vi "data_waypoint_ref.vi"() -> ()   [LabVIEW 2018] (continued)
"Y"=530235.061300714}, {"X"=175350.88993979365, "Y"=530235.1168702191}, {"X"=175350.93419405032, "Y"=530235.1720451514}, {"X"=175350.97797018028, "Y"=530235.2272858657}, {"X"=175351.0211706906, "Y"=530235.2819733487}, {"X"=175351.06420086315, "Y"=530235.3368710969}, {"X"=175351.1069546017, "Y"=530235.391745242}, {"X"=175351.14969397328, "Y"=530235.4471543846}, {"X"=175351.19290508452, "Y"=530235.5030349332}, {"X"=175351.23708086298, "Y"=530235.5592333905}, {"X"=175351.28094664667, "Y"=530235.6163428451}, {"X"=175351.32507018273, "Y"=530235.6737500923}, {"X"=175351.36946815113, "Y"=530235.7311032579}, {"X"=175351.4141272058, "Y"=530235.7883812926}, {"X"=175351.45875193508, "Y"=530235.845434128}, {"X"=175351.5033432786, "Y"=530235.9016790844}, {"X"=175351.5477972615, "Y"=530235.9573007046}, {"X"=175351.5920627689, "Y"=530236.0123890406}, {"X"=175351.63490704828, "Y"=530236.0676302855}, {"X"=175351.67720670445, "Y"=530236.1229175301}, {"X"=175351.71963278952, "Y"=530236.1781233831}, {"X"=175351.76294240737, "Y"=530236.2322667169}, {"X"=175351.80625901482, "Y"=530236.2860770716}, {"X"=175351.84902049394, "Y"=530236.3393729797}, {"X"=175351.89089530785, "Y"=530236.3929711628}, {"X"=175351.9331973055, "Y"=530236.4457479022}, {"X"=175351.97514771618, "Y"=530236.498248212}, {"X"=175352.01617310618, "Y"=530236.5512595625}, {"X"=175352.05664432573, "Y"=530236.6049850797}, {"X"=175352.09796583082, "Y"=530236.6580865675}, {"X"=175352.13995707338, "Y"=530236.7103159536}, {"X"=175352.18166292325, "Y"=530236.7621876963}, {"X"=175352.22252090828, "Y"=530236.813099689}, {"X"=175352.26255605364, "Y"=530236.8637288735}, {"X"=175352.30208352584, "Y"=530236.9137169486}, {"X"=175352.34150491114, "Y"=530236.9634744846}, {"X"=175352.38042420865, "Y"=530237.0135842154}, {"X"=175352.4199305173, "Y"=530237.0639053108}, {"X"=175352.45956587067, "Y"=530237.114131686}, {"X"=175352.49899166732, "Y"=530237.1641844318}, {"X"=175352.53829575534, "Y"=530237.2141165627}, {"X"=175352.5774806659, "Y"=530237.2632843519}, {"X"=175352.6156511215, "Y"=530237.3132742075}, {"X"=175352.6533883326, "Y"=530237.3629312733}, {"X"=175352.6910130333, "Y"=530237.4119815769}, {"X"=175352.72911552244, "Y"=530237.4611514483}, {"X"=175352.7674107072, "Y"=530237.5110854433}, {"X"=175352.80628102296, "Y"=530237.5626092828}, {"X"=175352.84566256969, "Y"=530237.6153813166}, {"X"=175352.886305737, "Y"=530237.6688455134}, {"X"=175352.92686425932, "Y"=530237.7224420327}, {"X"=175352.96628213656, "Y"=530237.776421486}, {"X"=175353.00479581486, "Y"=530237.8295612222}, {"X"=175353.04309125987, "Y"=530237.8813875283}, {"X"=175353.0805856114, "Y"=530237.9321951261}, {"X"=175353.1178263727, "Y"=530237.9820145867}, {"X"=175353.15486826623, "Y"=530238.031681473}, {"X"=175353.19223656916, "Y"=530238.0808956837}, {"X"=175353.22936573613, "Y"=530238.1307199139}, {"X"=175353.26626025818, "Y"=530238.1808755734}, {"X"=175353.3027933256, "Y"=530238.2313119823}, {"X"=175353.33960005036, "Y"=530238.2823335917}, {"X"=175353.37707444988, "Y"=530238.3338859645}, {"X"=175353.41547161504, "Y"=530238.386566564}, {"X"=175353.45446338505, "Y"=530238.4399313043}, {"X"=175353.49378934092, "Y"=530238.4939798436}, {"X"=175353.53226842728, "Y"=530238.5480086806}, {"X"=175353.57047974097, "Y"=530238.6019472994}, {"X"=175353.60875617847, "Y"=530238.6557414449}, {"X"=175353.6469764394, "Y"=530238.7094103412}, {"X"=175353.68457545002, "Y"=530238.7638723999}, {"X"=175353.72234228044, "Y"=530238.8184738057}, {"X"=175353.76045086328, "Y"=530238.8730198212}, {"X"=175353.79898426452, "Y"=530238.9271461678}, {"X"=175353.8375490814, "Y"=530238.9808107199}, {"X"=175353.8752460613, "Y"=530239.0342536401}, {"X"=175353.91189012938, "Y"=530239.0874910104}, {"X"=175353.94910051365, "Y"=530239.1393293964}, {"X"=175353.98627210603, "Y"=530239.1909281688}, {"X"=175354.02308637538, "Y"=530239.2430096754}, {"X"=175354.05967783305, "Y"=530239.2955291213}, {"X"=175354.09668178417, "Y"=530239.3488542204}, {"X"=175354.1341990515, "Y"=530239.4023320772}, {"X"=175354.17198692198, "Y"=530239.4562597376}, {"X"=175354.20951566947, "Y"=530239.5106276667}, {"X"=175354.24727854424, "Y"=530239.5653911263}, {"X"=175354.28528886437, "Y"=530239.6202604033}, {"X"=175354.3236916914, "Y"=530239.6751662572}, {"X"=175354.36217982642, "Y"=530239.7301650902}, {"X"=175354.401261916, "Y"=530239.784725996}, {"X"=175354.4399844256, "Y"=530239.8399039346}, {"X"=175354.47800392206, "Y"=530239.8951827234}, {"X"=175354.51573281956, "Y"=530239.9501405099}, {"X"=175354.55374814585, "Y"=530240.0043061222}, {"X"=175354.5920931261, "Y"=530240.0585195966}, {"X"=175354.6307848023, "Y"=530240.1125533618}, {"X"=175354.66938268108, "Y"=530240.1672211337}, {"X"=175354.70835670453, "Y"=530240.22178347}, {"X"=175354.74747454954, "Y"=530240.2767560309}, {"X"=175354.78668856682, "Y"=530240.3322011083}, {"X"=175354.82573295297, "Y"=530240.3880961786}, {"X"=175354.86442117963, "Y"=530240.4448679785}, {"X"=175354.90385480528, "Y"=530240.5017940709}, {"X"=175354.9438868584, "Y"=530240.5585985357}, {"X"=175354.98450460396, "Y"=530240.6151670938}, {"X"=175355.02560184867, "Y"=530240.6712336912}, {"X"=175355.0663030908, "Y"=530240.7269795968}, {"X"=175355.10590519384, "Y"=530240.7830661403}, {"X"=175355.1451417851, "Y"=530240.8386587655}, {"X"=175355.1843346686, "Y"=530240.8944490728}, {"X"=175355.22404374706, "Y"=530240.9501668296}, {"X"=175355.2643191493, "Y"=530241.0056886901}, {"X"=175355.30494895973, "Y"=530241.0609420296}, {"X"=175355.34536480953, "Y"=530241.1163314045}, {"X"=175355.38549545314, "Y"=530241.1717260601}, {"X"=175355.42590157175, "Y"=530241.2271199028}, {"X"=175355.466450924, "Y"=530241.2827253059}, {"X"=175355.50749417936, "Y"=530241.3382071704}, {"X"=175355.54871472975, "Y"=530241.3943377783}, {"X"=175355.5905385754, "Y"=530241.4498939218}, {"X"=175355.6317120192, "Y"=530241.5056695165}, {"X"=175355.6725872653, "Y"=530241.5612506543}, {"X"=175355.7131346146, "Y"=530241.6170791457}, {"X"=175355.7536999294, "Y"=530241.6726922737}, {"X"=175355.79431457655, "Y"=530241.7288135714}, {"X"=175355.83564892667, "Y"=530241.7844865855}, {"X"=175355.87750007684, "Y"=530241.8402923684}, {"X"=175355.9195047443, "Y"=530241.8958912657}, {"X"=175355.96087904507, "Y"=530241.9515952377}, {"X"=175356.0021839649, "Y"=530242.0072017458}, {"X"=175356.04336760036, "Y"=530242.0628308104}, {"X"=175356.08446281333, "Y"=530242.1185134072}, {"X"=175356.1253711881, "Y"=530242.1742165342}, {"X"=175356.16642529293, "Y"=530242.2294763982}, {"X"=175356.20768692662, "Y"=530242.2839210114}, {"X"=175356.24861907747, "Y"=530242.3386751397}, {"X"=175356.28909854963, "Y"=530242.3934161742}, {"X"=175356.3297216975, "Y"=530242.4482167154}, {"X"=175356.37073719004, "Y"=530242.5026975726}, {"X"=175356.4121149016, "Y"=530242.5571573845}, {"X"=175356.45343968744, "Y"=530242.6113920517}, {"X"=175356.4948522827, "Y"=530242.6656653044}, {"X"=175356.53583169985, "Y"=530242.7208310526}, {"X"=175356.57724413514, "Y"=530242.7765537826}, {"X"=175356.61908518994, "Y"=530242.8331442699}, {"X"=175356.66122786675, "Y"=530242.8895895861}, {"X"=175356.7031677672, "Y"=530242.9460588078}, {"X"=175356.74520092676, "Y"=530243.0017108984}, {"X"=175356.78699071577, "Y"=530243.0568376329}, {"X"=175356.82860514967, "Y"=530243.1110725575}, {"X"=175356.86955351502, "Y"=530243.1650197727}, {"X"=175356.90969446828, "Y"=530243.2182091132}, {"X"=175356.9490777895, "Y"=530243.2712996902}, {"X"=175356.98857629084, "Y"=530243.3234998218}, {"X"=175357.02793550797, "Y"=530243.375025569}, {"X"=175357.06710013995, "Y"=530243.4266473373}, {"X"=175357.10620575276, "Y"=530243.4780817132}, {"X"=175357.14540980468, "Y"=530243.5298554179}, {"X"=175357.18500684414, "Y"=530243.5818288475}, {"X"=175357.2246604417, "Y"=530243.6349596942}, {"X"=175357.2641467288, "Y"=530243.6890266448}, {"X"=175357.30388953027, "Y"=530243.7438730717}, {"X"=175357.34434687858, "Y"=530243.7989260455}, {"X"=175357.38561276108, "Y"=530243.853314052}, {"X"=175357.42714635562, "Y"=530243.9080741812}, {"X"=175357.46842059385, "Y"=530243.9631946698}, {"X"=175357.50957774406, "Y"=530244.0191612169}, {"X"=175357.55071779378, "Y"=530244.0753364675}, {"X"=175357.5918336218, "Y"=530244.1320090053}, {"X"=175357.63331725454, "Y"=530244.1881499484}, {"X"=175357.6750473695, "Y"=530244.2440715226}, {"X"=175357.7166139784, "Y"=530244.2995152301}, {"X"=175357.75781324354, "Y"=530244.3550454788}, {"X"=175357.79876509352, "Y"=530244.4101791265}, {"X"=175357.8395200305, "Y"=530244.4652223483}, {"X"=175357.88012770392, "Y"=530244.5204901953}, {"X"=175357.92098501846, "Y"=530244.5757073621}, {"X"=175357.96204256182, "Y"=530244.6303379341}, {"X"=175358.0031356214, "Y"=530244.6843968236}, {"X"=175358.04383856695, "Y"=530244.7389307731}, {"X"=175358.08452646548, "Y"=530244.7931695447}, {"X"=175358.12566475326, "Y"=530244.8472460592}, {"X"=175358.16694392514, "Y"=530244.9013388081}, {"X"=175358.20819046954, "Y"=530244.9557823667}, {"X"=175358.2494700914, "Y"=530245.0103279366}, {"X"=175358.29098381952, "Y"=530245.064361171}, {"X"=175358.33216177375, "Y"=530245.118073536}, {"X"=175358.3732513863, "Y"=530245.1718660723}, {"X"=175358.41425988183, "Y"=530245.2263869141}, {"X"=175358.45530746563, "Y"=530245.2806457151}, {"X"=175358.4961279473, "Y"=530245.3353901925}, {"X"=175358.53755439995, "Y"=530245.389565749}, {"X"=175358.57880946694, "Y"=530245.4429948742}, {"X"=175358.6194754227, "Y"=530245.4955001123}, {"X"=175358.65923557561, "Y"=530245.5475241211}, {"X"=175358.6986810228, "Y"=530245.5985601745}, {"X"=175358.73818095252, "Y"=530245.6497481184}, {"X"=175358.77788761366, "Y"=530245.7016557507}, {"X"=175358.81772277673, "Y"=530245.7538848643}, {"X"=175358.8581828618, "Y"=530245.8068668401}, {"X"=175358.89923729494, "Y"=530245.8601456174}, {"X"=175358.94051532645, "Y"=530245.9144559056}, {"X"=175358.9816894016, "Y"=530245.9692592768}, {"X"=175359.02267067126, "Y"=530246.024462766}, {"X"=175359.06317469152, "Y"=530246.0791293798}, {"X"=175359.10328494103, "Y"=530246.1330302408}, {"X"=175359.1426311365, "Y"=530246.1864572257}, {"X"=175359.18170182902, "Y"=530246.2389749364}, {"X"=175359.22067294916, "Y"=530246.2913686386}, {"X"=175359.26036426862, "Y"=530246.3431819814}, {"X"=175359.3002206982, "Y"=530246.3951147026}, {"X"=175359.33957727332, "Y"=530246.4472564398}, {"X"=175359.37847526275, "Y"=530246.4997835399}, {"X"=175359.41736539445, "Y"=530246.5517468553}, {"X"=175359.45611866727, "Y"=530246.6035596343}, {"X"=175359.49516651212, "Y"=530246.6552394703}, {"X"=175359.534532394, "Y"=530246.7066320259}, {"X"=175359.5738779074, "Y"=530246.7589269583}, {"X"=175359.61317105513, "Y"=530246.8120899559}, {"X"=175359.65284148513, "Y"=530246.8658334052}, {"X"=175359.6924238613, "Y"=530246.9197546942}, {"X"=175359.7321189642, "Y"=530246.9737555607}, {"X"=175359.7722131497, "Y"=530247.0267175318}, {"X"=175359.812302406, "Y"=530247.078607394}, {"X"=175359.8517182705, "Y"=530247.1301296569}, {"X"=175359.89077924602, "Y"=530247.180555317}, {"X"=175359.9290297936, "Y"=530247.2313018942}, {"X"=175359.96678072223, "Y"=530247.2823373973}, {"X"=175360.00470898786, "Y"=530247.3328329864}, {"X"=175360.04301417153, "Y"=530247.3831842932}, {"X"=175360.0812444498, "Y"=530247.4339664449}, {"X"=175360.11974357752, "Y"=530247.4852061785}, {"X"=175360.15889532102, "Y"=530247.5363762868}, {"X"=175360.19878413517, "Y"=530247.5878805108}, {"X"=175360.23892902656, "Y"=530247.6391142854}, {"X"=175360.278401387, "Y"=530247.6905731225}, {"X"=175360.31737113406, "Y"=530247.7419035878}, {"X"=175360.3562170554, "Y"=530247.7923964746}, {"X"=175360.39471564715, "Y"=530247.8425529867}, {"X"=175360.43373020628, "Y"=530247.8922584872}, {"X"=175360.47263689383, "Y"=530247.9426313309}, {"X"=175360.51171172748, "Y"=530247.9935541683}, {"X"=175360.55096069007, "Y"=530248.0452522838}, {"X"=175360.59049010673, "Y"=530248.0971371413}, {"X"=175360.63068016354, "Y"=530248.1486704462}, {"X"=175360.67107729564, "Y"=530248.2001354393}, {"X"=175360.71119287587, "Y"=530248.2510430022}, {"X"=175360.75040324742, "Y"=530248.3025725349}, {"X"=175360.78979999508, "Y"=530248.3545254847}, {"X"=175360.8304710297, "Y"=530248.4066589174}, {"X"=175360.87127768132, "Y"=530248.4591260182}, {"X"=175360.91191723972, "Y"=530248.5123017002}, {"X"=175360.9523743838, "Y"=530248.5657975603}, {"X"=175360.99262587648, "Y"=530248.618641429}, {"X"=175361.0330122471, "Y"=530248.6709654863}, {"X"=175361.0729788118, "Y"=530248.7224062232}, {"X"=175361.11191044463, "Y"=530248.7737323643}, {"X"=175361.1505965638, "Y"=530248.8241047515}, {"X"=175361.18968035345, "Y"=530248.8732595601}, {"X"=175361.22874977769, "Y"=530248.921748496}, {"X"=175361.26740235148, "Y"=530248.9697558712}, {"X"=175361.3060301731, "Y"=530249.0177799684}, {"X"=175361.34393528936, "Y"=530249.066737368}, {"X"=175361.38214647444, "Y"=530249.1170578811}, {"X"=175361.4216719192, "Y"=530249.1682002577}, {"X"=175361.46218246105, "Y"=530249.2199790122}, {"X"=175361.50222234274, "Y"=530249.2728556928}, {"X"=175361.54213471914, "Y"=530249.3257493963}, {"X"=175361.5823825225, "Y"=530249.3776443499}, {"X"=175361.62273221207, "Y"=530249.428344794}, {"X"=175361.6628429453, "Y"=530249.4785132093}, {"X"=175361.70243138418, "Y"=530249.528188167}, {"X"=175361.74098416534, "Y"=530249.578102579}, {"X"=175361.77956365625, "Y"=530249.6283642957}, {"X"=175361.81847626573, "Y"=530249.6783475681}, {"X"=175361.8581347175, "Y"=530249.7283353001}, {"X"=175361.8979152902, "Y"=530249.778284938}, {"X"=175361.93752073805, "Y"=530249.8283216615}, {"X"=175361.97688238163, "Y"=530249.8785866245}, {"X"=175362.0162104847, "Y"=530249.9285919806}, {"X"=175362.0553811717, "Y"=530249.978382486}, {"X"=175362.09459135542, "Y"=530250.0277489105}, {"X"=175362.1339222446, "Y"=530250.0774978804}, {"X"=175362.1736222086, "Y"=530250.1271469857}, {"X"=175362.21321350688, "Y"=530250.1768918592}, {"X"=175362.252683638, "Y"=530250.2270011243}, {"X"=175362.2924473459, "Y"=530250.2766389428}, {"X"=175362.33200780407, "Y"=530250.3264405108}, {"X"=175362.37099305278, "Y"=530250.376127239}, {"X"=175362.41009984864, "Y"=530250.4258801995}, {"X"=175362.44898119677, "Y"=530250.4751765631}, {"X"=175362.48782192072, "Y"=530250.52421334}, {"X"=175362.52699950442, "Y"=530250.5730404704}, {"X"=175362.5667985681, "Y"=530250.6220522263}, {"X"=175362.60660301094, "Y"=530250.6722892505}, {"X"=175362.64652048083, "Y"=530250.7230076215}, {"X"=175362.6858567776, "Y"=530250.7736921888}, {"X"=175362.7251310844, "Y"=530250.8240806081}, {"X"=175362.7639446701, "Y"=530250.8741296573}, {"X"=175362.8025109473, "Y"=530250.9235190699}, {"X"=175362.84085578495, "Y"=530250.9717071552}, {"X"=175362.87910314006, "Y"=530251.0198799929}, {"X"=175362.91751004552, "Y"=530251.0674885499}, {"X"=175362.95600635879, "Y"=530251.1153798591}, {"X"=175362.99435708468, "Y"=530251.1643636992}, {"X"=175363.0334184228, "Y"=530251.2137227969}, {"X"=175363.07259438004, "Y"=530251.2638029656}, {"X"=175363.11199823796, "Y"=530251.3139701424}, {"X"=175363.1513796253, "Y"=530251.364327171}, {"X"=175363.1906501197, "Y"=530251.4146268141}, {"X"=175363.22968945027, "Y"=530251.4646341368}, {"X"=175363.26866563145, "Y"=530251.5142531929}, {"X"=175363.3073697122, "Y"=530251.563214906}, {"X"=175363.34559084047, "Y"=530251.6127085537}, {"X"=175363.38380230192, "Y"=530251.6619292059}, {"X"=175363.42243679025, "Y"=530251.7104205436}, {"X"=175363.4610109799, "Y"=530251.7588898608}, {"X"=175363.49973307314, "Y"=530251.8073520857}, {"X"=175363.5383682305, "Y"=530251.8560709434}, {"X"=175363.57717002617, "Y"=530251.9048281554}, {"X"=175363.61560527026, "Y"=530251.9542412636}, {"X"=175363.65436447458, "Y"=530252.0032738473}, {"X"=175363.69337000587, "Y"=530252.0523334497}, {"X"=175363.7324087816, "Y"=530252.1018546579}, {"X"=175363.77137032332, "Y"=530252.1516169315}, {"X"=175363.81046026983, "Y"=530252.2025719273}, {"X"=175363.85010976103, "Y"=530252.253435373}, {"X"=175363.89048429485, "Y"=530252.3041590624}, {"X"=175363.9305881354, "Y"=530252.3547037531}, {"X"=175363.97065607106, "Y"=530252.4053872812}, {"X"=175364.0104260441, "Y"=530252.455955151}, {"X"=175364.05022246856, "Y"=530252.5055817852}, {"X"=175364.0895394326, "Y"=530252.5551210414}, {"X"=175364.12854528782, "Y"=530252.6042938508}, {"X"=175364.1669772529, "Y"=530252.6537979816}, {"X"=175364.2054922055, "Y"=530252.702908976}, {"X"=175364.24385568034, "Y"=530252.7514155437}, {"X"=175364.28218815473, "Y"=530252.799923314}, {"X"=175364.32078050665, "Y"=530252.848247191}, {"X"=175364.35987321084, "Y"=530252.8971334021}, {"X"=175364.39976063493, "Y"=530252.9472814032}, {"X"=175364.44051739766, "Y"=530252.9990649943}, {"X"=175364.48121062687, "Y"=530253.052132879}, {"X"=175364.5217449672, "Y"=530253.1050880281}, {"X"=175364.56172633727, "Y"=530253.1576607942}, {"X"=175364.60130530893, "Y"=530253.2095455242}, {"X"=175364.64039269785, "Y"=530253.2608368186}, {"X"=175364.67953891496, "Y"=530253.3116529188}, {"X"=175364.71831601113, "Y"=530253.3628541183}, {"X"=175364.75731318252, "Y"=530253.4135907482}, {"X"=175364.79603092565, "Y"=530253.4635879273}, {"X"=175364.8341888009, "Y"=530253.5129652326}, {"X"=175364.8714835971, "Y"=530253.5616292221}, {"X"=175364.90849024183, "Y"=530253.6105027163}, {"X"=175364.94563348373, "Y"=530253.6594390685}, {"X"=175364.98314331504, "Y"=530253.7089359304}, {"X"=175365.02100005752, "Y"=530253.7595272006}, {"X"=175365.05918145005, "Y"=530253.8114759818}, {"X"=175365.09803261896, "Y"=530253.864670273}, {"X"=175365.1369677881, "Y"=530253.9178143732}, {"X"=175365.175450904, "Y"=530253.9711551395}, {"X"=175365.2146263419, "Y"=530254.0234727964}, {"X"=175365.25404981908, "Y"=530254.0748962869}, {"X"=175365.29313406267, "Y"=530254.1257247813}, {"X"=175365.3311370293, "Y"=530254.1760414864}, {"X"=175365.36840857498, "Y"=530254.2258364942}, {"X"=175365.40494955413, "Y"=530254.2744971587}, {"X"=175365.44107322232, "Y"=530254.3225197739}, {"X"=175365.4766030218, "Y"=530254.3695064213}, {"X"=175365.51182505823, "Y"=530254.4166593428}, {"X"=175365.54752247653, "Y"=530254.4640172995}, {"X"=175365.58419388309, "Y"=530254.5115499632}, {"X"=175365.62093701866, "Y"=530254.5602788435}, {"X"=175365.65774631436, "Y"=530254.6098177265}, {"X"=175365.6950449408, "Y"=530254.6597857933}, {"X"=175365.73257001908, "Y"=530254.7099496393}, {"X"=175365.76995592058, "Y"=530254.7600772697}, {"X"=175365.80677752316, "Y"=530254.8101854757}, {"X"=175365.84416599848, "Y"=530254.8596838082}, {"X"=175365.88176222175, "Y"=530254.9096443404}, {"X"=175365.91953173553, "Y"=530254.9594944854}, {"X"=175365.9574402241, "Y"=530255.0090134849}, {"X"=175365.99470143978, "Y"=530255.0589117429}, {"X"=175366.03154062154, "Y"=530255.1089755029}, {"X"=175366.0680535847, "Y"=530255.1592533174}, {"X"=175366.10490100825, "Y"=530255.2091083997}, {"X"=175366.1418778741, "Y"=530255.2596034913}, {"X"=175366.1794578632, "Y"=530255.3106683819}, {"X"=175366.2173681856, "Y"=530255.3620142048}, {"X"=175366.25529422174, "Y"=530255.4138827252}, {"X"=175366.29256422166, "Y"=530255.465561172}, {"X"=175366.3293060358, "Y"=530255.517452049}, {"X"=175366.36565792985, "Y"=530255.5689833704}, {"X"=175366.40203412157, "Y"=530255.6200418209}, {"X"=175366.4388502521, "Y"=530255.6703997643}, {"X"=175366.47596965497, "Y"=530255.7205714668}, {"X"=175366.51282475406, "Y"=530255.770928185}, {"X"=175366.5496163633, "Y"=530255.821080876}, {"X"=175366.58622919343, "Y"=530255.8712851491}, {"X"=175366.62272470424, "Y"=530255.9216551357}, {"X"=175366.65895272506, "Y"=530255.9726318942}, {"X"=175366.69602994501, "Y"=530256.0244207871}, {"X"=175366.73390271078, "Y"=530256.0771507177}, {"X"=175366.77233000507, "Y"=530256.1316958538}, {"X"=175366.81173351035, "Y"=530256.1868696233}, {"X"=175366.8519770966, "Y"=530256.2427678755}, {"X"=175366.8918884384, "Y"=530256.2989401333}, {"X"=175366.93135789846, "Y"=530256.3554544192}, {"X"=175366.9706897959, "Y"=530256.4115784413}, {"X"=175367.01058779864, "Y"=530256.4677340913}, {"X"=175367.05065983246, "Y"=530256.5246328339}, {"X"=175367.09101690596, "Y"=530256.5811689214}, {"X"=175367.1310731591, "Y"=530256.6375227704}, {"X"=175367.17083612958, "Y"=530256.6932448632}, {"X"=175367.21025581684, "Y"=530256.7481999461}, {"X"=175367.2492354851, "Y"=530256.8023261506}, {"X"=175367.287581066, "Y"=530256.8564975066}, {"X"=175367.32615449073, "Y"=530256.910735893}, {"X"=175367.3651370734, "Y"=530256.9652505389}, {"X"=175367.40405244404, "Y"=530257.0192004658}, {"X"=175367.44224889282, "Y"=530257.0729627243}, {"X"=175367.48063509667, "Y"=530257.1270928971}, {"X"=175367.5193307458, "Y"=530257.1810268238}, {"X"=175367.55835376275, "Y"=530257.2354370258}, {"X"=175367.59777806984, "Y"=530257.2904586872}, {"X"=175367.63832748993, "Y"=530257.3464415018}, {"X"=175367.67939942481, "Y"=530257.4029932447}, {"X"=175367.7207491782, "Y"=530257.4600391674}, {"X"=175367.7617005033, "Y"=530257.5171439771}, {"X"=175367.80307118673, "Y"=530257.5743796235}, {"X"=175367.84486851882, "Y"=530257.6312133558}, {"X"=175367.88690845872, "Y"=530257.6877145241}, {"X"=175367.92825091735, "Y"=530257.7446905482}, {"X"=175367.9699223432, "Y"=530257.8011817061}, {"X"=175368.01151293772, "Y"=530257.8572957474}, {"X"=175368.05314487906, "Y"=530257.9130123383}, {"X"=175368.09419173302, "Y"=530257.9685697247}, {"X"=175368.13502857919, "Y"=530258.0240999819}, {"X"=175368.17578947498, "Y"=530258.0794073816}, {"X"=175368.21706993572, "Y"=530258.1336810826}, {"X"=175368.2580036735, "Y"=530258.1878248417}, {"X"=175368.29871781138, "Y"=530258.2416928933}, {"X"=175368.33960146687, "Y"=530258.29567476}, {"X"=175368.38056272513, "Y"=530258.349538754}, {"X"=175368.42160467047, "Y"=530258.403431366}, {"X"=175368.46324653408, "Y"=530258.4574065608}, {"X"=175368.50493600065, "Y"=530258.5113039257}, {"X"=175368.546039586, "Y"=530258.5653739354}, {"X"=175368.58627301786, "Y"=530258.619636295}, {"X"=175368.62661766922, "Y"=530258.6737673621}, {"X"=175368.66737663423, "Y"=530258.7275187485}, {"X"=175368.707789486, "Y"=530258.7819492777}, {"X"=175368.74817281184, "Y"=530258.8368815499}, {"X"=175368.78905969212, "Y"=530258.8922607239}, {"X"=175368.83060171016, "Y"=530258.9472239888}, {"X"=175368.87236381875, "Y"=530259.0017271258}, {"X"=175368.91362172773, "Y"=530259.0555647215}, {"X"=175368.9541187612, "Y"=530259.1088041244}, {"X"=175368.99351905257, "Y"=530259.161693824}, {"X"=175369.03251394143, "Y"=530259.2140797316}, {"X"=175369.07165795774, "Y"=530259.2668725194}, {"X"=175369.1116919916, "Y"=530259.3202020752}, {"X"=175369.1522712206, "Y"=530259.3739828493}, {"X"=175369.19244677763, "Y"=530259.4275450595}, {"X"=175369.2315454748, "Y"=530259.4811925745}, {"X"=175369.27035327113, "Y"=530259.5341139864}, {"X"=175369.30912567972, "Y"=530259.5858479531}, {"X"=175369.34761534786, "Y"=530259.637222049}, {"X"=175369.38570391198, "Y"=530259.6883464997}, {"X"=175369.4236531108, "Y"=530259.7393714729}, {"X"=175369.4617789277, "Y"=530259.7896123657}, {"X"=175369.49993611278, "Y"=530259.8390751553}, {"X"=175369.53771359075, "Y"=530259.8880362958}, {"X"=175369.57511864332, "Y"=530259.9371627924}, {"X"=175369.61242632216, "Y"=530259.9872129811}, {"X"=175369.65026476423, "Y"=530260.0379253004}, {"X"=175369.68844804208, "Y"=530260.0899329198}, {"X"=175369.72774864096, "Y"=530260.1420593341}, {"X"=175369.76747697193, "Y"=530260.1944530737}, {"X"=175369.80690045215, "Y"=530260.2470996501}, {"X"=175369.84600582987, "Y"=530260.2994086567}, {"X"=175369.8855787249, "Y"=530260.3516585723}, {"X"=175369.92548969664, "Y"=530260.4038098247}, {"X"=175369.96521553188, "Y"=530260.4568606102}, {"X"=175370.0048233524, "Y"=530260.5098418208}, {"X"=175370.04435833584, "Y"=530260.5630540976}, {"X"=175370.08360233658, "Y"=530260.6155147478}, {"X"=175370.12268043496, "Y"=530260.6666828998}, {"X"=175370.161077391, "Y"=530260.7169574014}, {"X"=175370.1988345409, "Y"=530260.7665367983}, {"X"=175370.23621340372, "Y"=530260.8160973303}, {"X"=175370.2741603868, "Y"=530260.8651700723}, {"X"=175370.31198308783, "Y"=530260.9147526048}, {"X"=175370.3494809023, "Y"=530260.9653027819}, {"X"=175370.38678381703, "Y"=530261.0161443175}, {"X"=175370.42433720775, "Y"=530261.0678208391}, {"X"=175370.4626341092, "Y"=530261.1193120438}, {"X"=175370.50168795633, "Y"=530261.1715712609}, {"X"=175370.54076009642, "Y"=530261.2252288469}, {"X"=175370.58048902013, "Y"=530261.279631433}, {"X"=175370.62107124308, "Y"=530261.333832843}, {"X"=175370.66210860672, "Y"=530261.3879840766}, {"X"=175370.70264565348, "Y"=530261.4421856187}, {"X"=175370.74249817466, "Y"=530261.4961483381}, {"X"=175370.78169428193, "Y"=530261.5497933521}, {"X"=175370.82119589235, "Y"=530261.6028059552}, {"X"=175370.8604972166, "Y"=530261.6560855159}, {"X"=175370.89999125095, "Y"=530261.7092335463}, {"X"=175370.93876096676, "Y"=530261.7621650669}, {"X"=175370.97771263926, "Y"=530261.8146221417}, {"X"=175371.01739352918, "Y"=530261.8662513338}, {"X"=175371.057154059, "Y"=530261.9175528833}, {"X"=175371.09605709632, "Y"=530261.9691366423}, {"X"=175371.13461257404, "Y"=530262.0218090902}, {"X"=175371.17493162048, "Y"=530262.074476341}, {"X"=175371.2161687712, "Y"=530262.1281930344}, {"X"=175371.2574986481, "Y"=530262.1824155508}, {"X"=175371.29896848748, "Y"=530262.2372436394}, {"X"=175371.34017383057, "Y"=530262.2927928045}, {"X"=175371.38163837852, "Y"=530262.3479305593}, {"X"=175371.4233859332, "Y"=530262.4026168778}, {"X"=175371.4653806578, "Y"=530262.457616558}, {"X"=175371.50709616198, "Y"=530262.5134505647}, {"X"=175371.5492311775, "Y"=530262.5688660291}, {"X"=175371.59135206408, "Y"=530262.6242970738}, {"X"=175371.63361993022, "Y"=530262.6797065984}, {"X"=175371.67533013487, "Y"=530262.7352465111}, {"X"=175371.7166030467, "Y"=530262.7908820468}, {"X"=175371.7576439664, "Y"=530262.846846788}, {"X"=175371.79961031346, "Y"=530262.9018365643}, {"X"=175371.8417403082, "Y"=530262.9558502925}, {"X"=175371.88340146284, "Y"=530263.0091728515}, {"X"=175371.92439824372, "Y"=530263.0615795128}, {"X"=175371.96503316762, "Y"=530263.1135310883}, {"X"=175372.0052249805, "Y"=530263.1648058448}, {"X"=175372.04496494954, "Y"=530263.216047527}, {"X"=175372.08486382675, "Y"=530263.267409716}, {"X"=175372.12527531054, "Y"=530263.3195872516}, {"X"=175372.16591554228, "Y"=530263.3718373646}, {"X"=175372.20672269005, "Y"=530263.4245209418}, {"X"=175372.24767576595, "Y"=530263.4771275077}, {"X"=175372.28965336786, "Y"=530263.5290240761}, {"X"=175372.33110264182, "Y"=530263.5816868937}, {"X"=175372.3726853523, "Y"=530263.6348432075}, {"X"=175372.4151099726, "Y"=530263.6881424303}, {"X"=175372.45798269208, "Y"=530263.7411051576}, {"X"=175372.50007205043, "Y"=530263.7942555395}, {"X"=175372.5416247459, "Y"=530263.8474474571}, {"X"=175372.5829580622, "Y"=530263.9010406794}, {"X"=175372.62484024334, "Y"=530263.9542238587}, {"X"=175372.66669413337, "Y"=530264.0071252142}, {"X"=175372.70904192966, "Y"=530264.0599052535}, {"X"=175372.75097860975, "Y"=530264.112345775}, {"X"=175372.7924628684, "Y"=530264.1645578903}, {"X"=175372.8333104372, "Y"=530264.2162313784}, {"X"=175372.8738449646, "Y"=530264.2680833666}, {"X"=175372.91441410081, "Y"=530264.319957451}, {"X"=175372.9557862025, "Y"=530264.3719834397}, {"X"=175372.99767016945, "Y"=530264.4239701862}, {"X"=175373.03924414562, "Y"=530264.4765704875}, {"X"=175373.0804756962, "Y"=530264.529296102}, {"X"=175373.12245933426, "Y"=530264.5811404951}, {"X"=175373.1641074646, "Y"=530264.6327539145}, {"X"=175373.2048067197, "Y"=530264.6842968779}, {"X"=175373.245243158, "Y"=530264.7356275225}, {"X"=175373.28613031158, "Y"=530264.7872098872}, {"X"=175373.3268719919, "Y"=530264.8396239675}, {"X"=175373.36816244232, "Y"=530264.8921995794}, {"X"=175373.40948345076, "Y"=530264.9443233894}, {"X"=175373.45060314657, "Y"=530264.9963656624}, {"X"=175373.49133239881, "Y"=530265.0475689222}, {"X"=175373.53206551704, "Y"=530265.0985812743}, {"X"=175373.5723972954, "Y"=530265.1501674973}, {"X"=175373.6127379377, "Y"=530265.2029590018}, {"X"=175373.65307959612, "Y"=530265.2560956681}, {"X"=175373.6935509451, "Y"=530265.3090554855}, {"X"=175373.73412274377, "Y"=530265.3609340055}, {"X"=175373.7750503279, "Y"=530265.4118103823}, {"X"=175373.8156763603, "Y"=530265.4625544671}, {"X"=175373.85636513907, "Y"=530265.512649098}, {"X"=175373.8966237603, "Y"=530265.5631567544}, {"X"=175373.9368359794, "Y"=530265.6141495564}, {"X"=175373.97664394762, "Y"=530265.6659315486}, {"X"=175374.01652882574, "Y"=530265.7176611514}, {"X"=175374.0558253849, "Y"=530265.7696377665}, {"X"=175374.09546728528, "Y"=530265.8215756294}, {"X"=175374.1352996199, "Y"=530265.8735107117}, {"X"=175374.1753605969, "Y"=530265.9263862808}, {"X"=175374.21554098636, "Y"=530265.9792048966}, {"X"=175374.25634345112, "Y"=530266.0321115775}, {"X"=175374.29684755186, "Y"=530266.0847660915}, {"X"=175374.3370072678, "Y"=530266.1368822271}, {"X"=175374.37684985562, "Y"=530266.1883899836}, {"X"=175374.41664284474, "Y"=530266.2401997693}, {"X"=175374.45623583646, "Y"=530266.2926760602}, {"X"=175374.4957903801, "Y"=530266.3453322599}, {"X"=175374.53494277128, "Y"=530266.3985856391}, {"X"=175374.5738609444, "Y"=530266.4514124128}, {"X"=175374.61273645412, "Y"=530266.5035878264}, {"X"=175374.6511642197, "Y"=530266.5553183937}, {"X"=175374.68891586334, "Y"=530266.6066558418}, {"X"=175374.72739777548, "Y"=530266.6569223469}, {"X"=175374.7656299184, "Y"=530266.7065947026}, {"X"=175374.80313963493, "Y"=530266.7566920433}, {"X"=175374.8399778119, "Y"=530266.8064484142}, {"X"=175374.8766657008, "Y"=530266.8563062254}, {"X"=175374.91344849125, "Y"=530266.9059040511}, {"X"=175374.95023190015, "Y"=530266.9560135192}, {"X"=175374.98740198716, "Y"=530267.0068876502}, {"X"=175375.02601149524, "Y"=530267.0580716352}, {"X"=175375.06553802377, "Y"=530267.1114426706}, {"X"=175375.10591067414, "Y"=530267.1669876481}, {"X"=175375.146517546, "Y"=530267.2238637658}, {"X"=175375.1877406851, "Y"=530267.2809611515}, {"X"=175375.22830013547, "Y"=530267.3382780246}, {"X"=175375.26785239112, "Y"=530267.3949719046}, {"X"=175375.30721058228, "Y"=530267.4504355218}, {"X"=175375.34715167427, "Y"=530267.5053180757}, {"X"=175375.38706773933, "Y"=530267.5595225785}, {"X"=175375.4267418654, "Y"=530267.613685621}, {"X"=175375.46535510637, "Y"=530267.6676442431}, {"X"=175375.50396058234, "Y"=530267.7216716999}, {"X"=175375.54284507962, "Y"=530267.7750990131}, {"X"=175375.58147326022, "Y"=530267.8287157561}, {"X"=175375.61925587003, "Y"=530267.8830519565}, {"X"=175375.6576886122, "Y"=530267.9376803568}, {"X"=175375.69664500767, "Y"=530267.9926623688}, {"X"=175375.73603756493, "Y"=530268.0480681743}, {"X"=175375.77532893803, "Y"=530268.1040047903}, {"X"=175375.81435740308, "Y"=530268.1602995562}, {"X"=175375.85262212646, "Y"=530268.2171293042}, {"X"=175375.89158039243, "Y"=530268.2739503484}, {"X"=175375.93173150255, "Y"=530268.330970986}, {"X"=175375.97191079802, "Y"=530268.3882379278}, {"X"=175376.01228297348, "Y"=530268.4463333681}, {"X"=175376.05265943654, "Y"=530268.5043810724}, {"X"=175376.09293965067, "Y"=530268.562530056}, {"X"=175376.13402299516, "Y"=530268.6205878863}, {"X"=175376.17550761972, "Y"=530268.6789541855}, {"X"=175376.2171191087, "Y"=530268.7382901298}, {"X"=175376.25857909265, "Y"=530268.798215855}, {"X"=175376.30063365336, "Y"=530268.8576137554}, {"X"=175376.34250984906, "Y"=530268.9169023044}, {"X"=175376.38375533113, "Y"=530268.9761782852}, {"X"=175376.4239993277, "Y"=530269.0352652095}, {"X"=175376.46462206956, "Y"=530269.0942278227}, {"X"=175376.5061171255, "Y"=530269.1522278391}, {"X"=175376.5475091983, "Y"=530269.20984859}, {"X"=175376.58769639168, "Y"=530269.2676948581}, {"X"=175376.62757688668, "Y"=530269.3254665607}, {"X"=175376.667320457, "Y"=530269.3824628744}, {"X"=175376.70731428557, "Y"=530269.4393174993}, {"X"=175376.74719239495, "Y"=530269.495980459}, {"X"=175376.7866007532, "Y"=530269.5537480027}, {"X"=175376.82704140185, "Y"=530269.6116368113}, {"X"=175376.86867427992, "Y"=530269.6692157873}, {"X"=175376.91032201465, "Y"=530269.7264251373}, {"X"=175376.9512818232, "Y"=530269.7837452792}, {"X"=175376.99105095697, "Y"=530269.8410012267}, {"X"=175377.02996204546, "Y"=530269.8986514817}, {"X"=175377.06897030905, "Y"=530269.9562137703}, {"X"=175377.1089557823, "Y"=530270.0135423321}, {"X"=175377.14928842592, "Y"=530270.0708510028}, {"X"=175377.18985192844, "Y"=530270.1274475757}, {"X"=175377.2301206264, "Y"=530270.1834967455}, {"X"=175377.2706423454, "Y"=530270.2388393001}, {"X"=175377.31043959537, "Y"=530270.2942139549}, {"X"=175377.34961013673, "Y"=530270.3497336272}, {"X"=175377.38805029093, "Y"=530270.4062842885}, {"X"=175377.42698760645, "Y"=530270.4629167287}, {"X"=175377.4664671266, "Y"=530270.5195853052}, {"X"=175377.50645504915, "Y"=530270.5753411908}, {"X"=175377.5459466516, "Y"=530270.6313005314}, {"X"=175377.58575752817, "Y"=530270.6876951077}, {"X"=175377.62575899236, "Y"=530270.7447406121}, {"X"=175377.66585884744, "Y"=530270.8024117845}, {"X"=175377.70568216513, "Y"=530270.8603246126}, {"X"=175377.74558738028, "Y"=530270.9180740495}, {"X"=175377.7855966506, "Y"=530270.974763265}, {"X"=175377.82569728378, "Y"=530271.0302924092}, {"X"=175377.86556871625, "Y"=530271.084692392}, {"X"=175377.90532123862, "Y"=530271.1393202449}, {"X"=175377.94501325546, "Y"=530271.1944565923}, {"X"=175377.98486513883, "Y"=530271.2503405145}, {"X"=175378.02435570536, "Y"=530271.3062510273}, {"X"=175378.06409336728, "Y"=530271.3621497148}, {"X"=175378.103309077, "Y"=530271.4176703686}, {"X"=175378.14220560313, "Y"=530271.473087634}, {"X"=175378.1814429543, "Y"=530271.5284373041}, {"X"=175378.22134028416, "Y"=530271.5838127786}, {"X"=175378.26121354155, "Y"=530271.6397365938}, {"X"=175378.30082891998, "Y"=530271.695920876}, {"X"=175378.34050395305, "Y"=530271.7519096485}, {"X"=175378.38047696327, "Y"=530271.8074180826}, {"X"=175378.42039218737, "Y"=530271.8628545483}, {"X"=175378.46029272696, "Y"=530271.9181179173}, {"X"=175378.50024812756, "Y"=530271.973962691}, {"X"=175378.54103024217, "Y"=530272.0296030378}, {"X"=175378.58160302788, "Y"=530272.0854482147}, {"X"=175378.6219478474, "Y"=530272.1405826434}, {"X"=175378.66133265817, "Y"=530272.1948741865}, {"X"=175378.70041345863, "Y"=530272.2478991648}, {"X"=175378.73875308977, "Y"=530272.3003991435}, {"X"=175378.7769726777, "Y"=530272.3530437571}, {"X"=175378.81478900305, "Y"=530272.4059093122}, {"X"=175378.85344642977, "Y"=530272.4595459604}, {"X"=175378.8927827093, "Y"=530272.5129997034}, {"X"=175378.9328368426, "Y"=530272.5662793056}, {"X"=175378.97299077566, "Y"=530272.619159064}, {"X"=175379.01313879451, "Y"=530272.6724361693}, {"X"=175379.05281503018, "Y"=530272.7267301857}, {"X"=175379.09275090517, "Y"=530272.7819634884}, {"X"=175379.13273609988, "Y"=530272.8380035125}, {"X"=175379.17377965036, "Y"=530272.8933911546}, {"X"=175379.21499514012, "Y"=530272.9488104766}, {"X"=175379.25621501883, "Y"=530273.0033163701}, {"X"=175379.2960237182, "Y"=530273.0580761392}, {"X"=175379.33575262167, "Y"=530273.1128117243}, {"X"=175379.3756350914, "Y"=530273.1676578454}, {"X"=175379.41577269154, "Y"=530273.222211321}, {"X"=175379.45561149748, "Y"=530273.2769687815}, {"X"=175379.49584439732, "Y"=530273.3307983498}, {"X"=175379.53572220702, "Y"=530273.3837610537}, {"X"=175379.57504594701, "Y"=530273.4362681268}, {"X"=175379.61395791481, "Y"=530273.4879118324}, {"X"=175379.653285014, "Y"=530273.5397552007}, {"X"=175379.69188306064, "Y"=530273.5924819438}, {"X"=175379.73056062285, "Y"=530273.6460419565}, {"X"=175379.76959291293, "Y"=530273.6994422176}, {"X"=175379.8094673134, "Y"=530273.7524515456}, {"X"=175379.8491786922, "Y"=530273.8051483744}, {"X"=175379.88896082636, "Y"=530273.8581091418}, {"X"=175379.9291784505, "Y"=530273.9121673888}, {"X"=175379.97054167185, "Y"=530273.9666229206}, {"X"=175380.01182172928, "Y"=530274.0226169619}, {"X"=175380.05318232844, "Y"=530274.079491995}, {"X"=175380.09513207295, "Y"=530274.1364019196}, {"X"=175380.13819652947, "Y"=530274.1925460887}, {"X"=175380.18149366078, "Y"=530274.2491956674}, {"X"=175380.2250484434, "Y"=530274.3055070925}, {"X"=175380.26838144008, "Y"=530274.3623041774}, {"X"=175380.31188147655, "Y"=530274.4186745853}, {"X"=175380.3549409229, "Y"=530274.4749230964}, {"X"=175380.3972649774, "Y"=530274.5308053015}, {"X"=175380.43836973322, "Y"=530274.5862271729}, {"X"=175380.47931384272, "Y"=530274.6406384385}, {"X"=175380.5204471117, "Y"=530274.694614081}, {"X"=175380.56209510507, "Y"=530274.748920056}, {"X"=175380.60371871642, "Y"=530274.8033692753}, {"X"=175380.6451534636, "Y"=530274.8583540027}, {"X"=175380.68621689494, "Y"=530274.91297912}, {"X"=175380.72710987853, "Y"=530274.9677778766}, {"X"=175380.76810750342, "Y"=530275.0226162815}, {"X"=175380.80994694738, "Y"=530275.0778672938}, {"X"=175380.85239067252, "Y"=530275.1334805603}, {"X"=175380.89503053552, "Y"=530275.1901265308}, {"X"=175380.9377349384, "Y"=530275.246731244}, {"X"=175380.9805978658, "Y"=530275.3030247326}, {"X"=175381.0230490275, "Y"=530275.3587578452}, {"X"=175381.06513342983, "Y"=530275.4135730725}, {"X"=175381.10631238978, "Y"=530275.4686295863}, {"X"=175381.14743795973, "Y"=530275.5233022464}, {"X"=175381.18891169218, "Y"=530275.5779927488}, {"X"=175381.23041948982, "Y"=530275.6325200024}, {"X"=175381.27197850702, "Y"=530275.6875975949}, {"X"=175381.3141971989, "Y"=530275.7425955562}, {"X"=175381.35612077633, "Y"=530275.7987464201}, {"X"=175381.39866254883, "Y"=530275.8545702754}, {"X"=175381.44144096706, "Y"=530275.9110449206}, {"X"=175381.48396489912, "Y"=530275.9674281975}, {"X"=175381.52566846483, "Y"=530276.0237661658}, {"X"=175381.56639495818, "Y"=530276.0791813901}, {"X"=175381.60614632058, "Y"=530276.1337315745}, {"X"=175381.64565829624, "Y"=530276.1873035681}, {"X"=175381.68537671026, "Y"=530276.2408927118}, {"X"=175381.72567720927, "Y"=530276.2954279619}, {"X"=175381.76592636586, "Y"=530276.3505771153}, {"X"=175381.8065536897, "Y"=530276.4066074943}, {"X"=175381.84723761232, "Y"=530276.4623069686}, {"X"=175381.8881185681, "Y"=530276.5175375018}, {"X"=175381.92892906343, "Y"=530276.5717005575}, {"X"=175381.96981449414, "Y"=530276.6260454104}, {"X"=175382.0109063195, "Y"=530276.6806926475}, {"X"=175382.05228986236, "Y"=530276.7360426767}, {"X"=175382.09401500106, "Y"=530276.7918878068}, {"X"=175382.13590830663, "Y"=530276.848290703}, {"X"=175382.17683812688, "Y"=530276.9053778878}, {"X"=175382.21736197197, "Y"=530276.9623663815}, {"X"=175382.25794670594, "Y"=530277.0195777777}, {"X"=175382.299110183, "Y"=530277.076300242}, {"X"=175382.3405598369, "Y"=530277.1330462806}, {"X"=175382.3816216344, "Y"=530277.1898323065}, {"X"=175382.42177914153, "Y"=530277.246647631}, {"X"=175382.4623105062, "Y"=530277.3016794228}, {"X"=175382.50294386526, "Y"=530277.3558518823}, {"X"=175382.54306338512, "Y"=530277.4093932352}, {"X"=175382.58212770906, "Y"=530277.4634571102}, {"X"=175382.62030600384, "Y"=530277.5183382287}, {"X"=175382.65887284116, "Y"=530277.5734135413}, {"X"=175382.69841257622, "Y"=530277.6285958623}, {"X"=175382.73787164403, "Y"=530277.6837573361}, {"X"=175382.77683788392, "Y"=530277.7388048348}, {"X"=175382.81560297194, "Y"=530277.7935244082}, {"X"=175382.85500985917, "Y"=530277.8484130106}, {"X"=175382.89468581765, "Y"=530277.9029312362}, {"X"=175382.93342362894, "Y"=530277.9580138144}, {"X"=175382.97016422707, "Y"=530278.0137726283}, {"X"=175383.00719641265, "Y"=530278.0689867527}, {"X"=175383.04524049233, "Y"=530278.1234110076}, {"X"=175383.08446525745, "Y"=530278.177516587}, {"X"=175383.12400785997, "Y"=530278.2324713808}, {"X"=175383.16341338272, "Y"=530278.2884021463}, {"X"=175383.20321088587, "Y"=530278.3450931216}, {"X"=175383.24388467334, "Y"=530278.4018691962}, {"X"=175383.28416762798, "Y"=530278.46038113}, {"X"=175383.32348511857, "Y"=530278.5201078751}, {"X"=175383.36322165257, "Y"=530278.5798589126}, {"X"=175383.40385465274, "Y"=530278.6390279633}, {"X"=175383.44465535972, "Y"=530278.6989001713}, {"X"=175383.4862341692, "Y"=530278.75830284}, {"X"=175383.52822093136, "Y"=530278.8175722327}, {"X"=175383.56995807827, "Y"=530278.8769011825}, {"X"=175383.61148408483, "Y"=530278.9361197695}, {"X"=175383.65323525056, "Y"=530278.9944953114}, {"X"=175383.69421530858, "Y"=530279.0530074155}, {"X"=175383.7350554744, "Y"=530279.111541019}, {"X"=175383.77542995836, "Y"=530279.1704555652}, {"X"=175383.8157298488, "Y"=530279.2293070713}, {"X"=175383.8559401721, "Y"=530279.2881233235}, {"X"=175383.89695070562, "Y"=530279.3461569902}, {"X"=175383.93826252603, "Y"=530279.4039311717}, {"X"=175383.97949878522, "Y"=530279.4619153388}, {"X"=175384.02036026714, "Y"=530279.5201691986}, {"X"=175384.06054778706, "Y"=530279.5790632094}, {"X"=175384.10039149693, "Y"=530279.6382146104}, {"X"=175384.14101006766, "Y"=530279.6973004678}, {"X"=175384.1822571442, "Y"=530279.7559505224}, {"X"=175384.22384488, "Y"=530279.8141767163}, {"X"=175384.26575571846, "Y"=530279.8720312649}, {"X"=175384.30757643149, "Y"=530279.9302634323}, {"X"=175384.34938070193, "Y"=530279.988026178}, {"X"=175384.39056756336, "Y"=530280.0457807535}, {"X"=175384.4300316461, "Y"=530280.1038567104}, {"X"=175384.46858665868, "Y"=530280.1612416819}, {"X"=175384.5074643027, "Y"=530280.2174947566}, {"X"=175384.54749630456, "Y"=530280.2726090478}, {"X"=175384.586673461, "Y"=530280.3276992185}, {"X"=175384.62548891825, "Y"=530280.3817849228}, {"X"=175384.66357065516, "Y"=530280.4351669155}, {"X"=175384.70142916602, "Y"=530280.4873442599}, {"X"=175384.7383800607, "Y"=530280.538421075}, {"X"=175384.77384348479, "Y"=530280.5882103939}, {"X"=175384.80759560052, "Y"=530280.6358982379}, {"X"=175384.8404099675, "Y"=530280.6812770056}, {"X"=175384.87250879448, "Y"=530280.7243071992}, {"X"=175384.90436964578, "Y"=530280.7647299246}, {"X"=175384.93436790677, "Y"=530280.80311488}, {"X"=175384.9616378935, "Y"=530280.8381638632}, {"X"=175384.9850736076, "Y"=530280.8648757731}, {"X"=175385.00324402758, "Y"=530280.8833868961}, {"X"=175385.0150459357, "Y"=530280.8944529634}, {"X"=175385.02297698648, "Y"=530280.9010033109}, {"X"=175385.02939790592, "Y"=530280.9042851299}, {"X"=175385.03577591613, "Y"=530280.9056281495}, {"X"=175385.04157625238, "Y"=530280.9066199363}, {"X"=175385.04734175224, "Y"=530280.9069115034}, {"X"=175385.0522705122, "Y"=530280.9070113084}, {"X"=175385.05647557072, "Y"=530280.9068024849}, {"X"=175385.06001046783, "Y"=530280.9061183934}, {"X"=175385.06346903727, "Y"=530280.9044811573}, {"X"=175385.06641534183, "Y"=530280.9021439983}, {"X"=175385.06904727407, "Y"=530280.8992328586}, {"X"=175385.0711258982, "Y"=530280.896123573}, {"X"=175385.0733705323, "Y"=530280.8925376674}, {"X"=175385.0755269345, "Y"=530280.8887688976}, {"X"=175385.07764847262, "Y"=530280.8848914615}, {"X"=175385.07942518912, "Y"=530280.8812292453}, {"X"=175385.08167830165, "Y"=530280.8775145715}, {"X"=175385.08414133126, "Y"=530280.8740967229}, {"X"=175385.08691378706, "Y"=530280.871078623}]
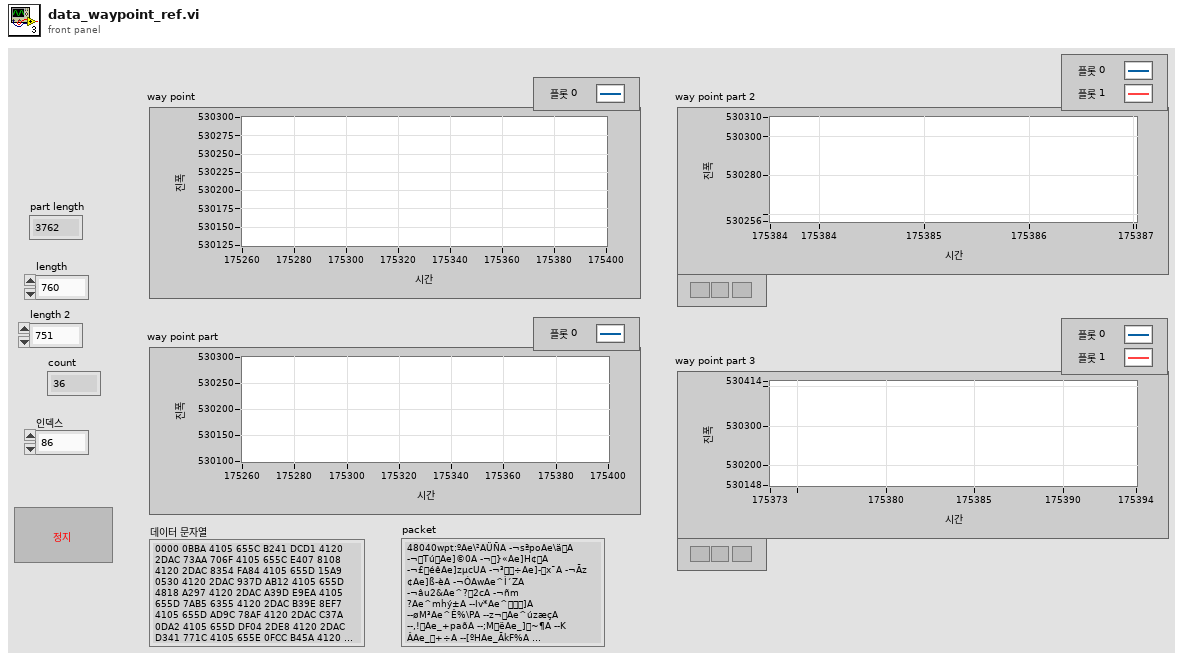
[diagram p1: front panel]
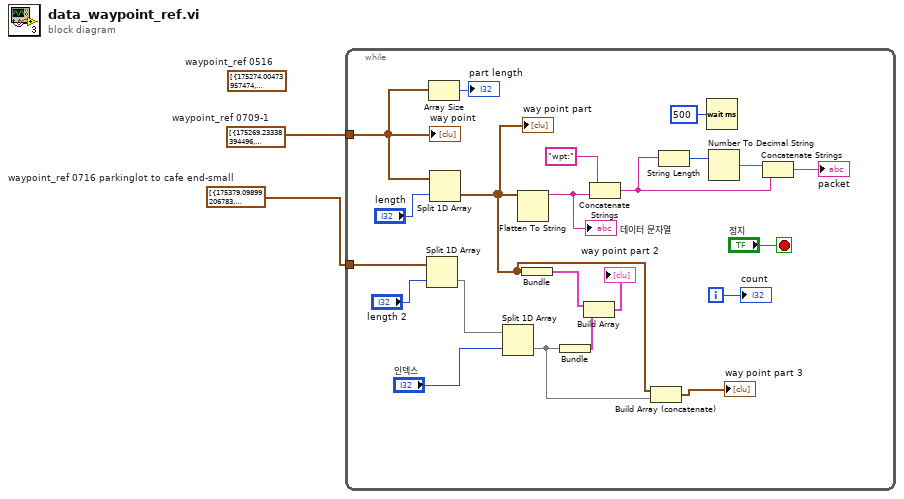
[diagram p0: block diagram]
diagram:
